vi "Read Method.vi"(11 "Filter in":refnum<class "Filter.lvclass">) -> (2 "Method":T1, 3 "Filter out":refnum<class "Filter.lvclass">)   [LabVIEW 2018, in "GLog.lvlib" / "Filter.lvclass"]
uses:
  Filter.lvclass
  Aggregation Method.ctl
  Filter.lvclass/Filter.ctl
  GLog.lvlib
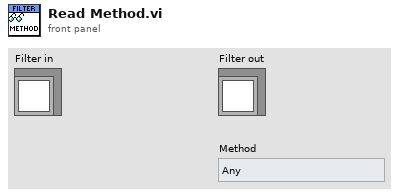
[diagram p1: front panel]
types:
  T1 = typedef "GLog.lvlib/Aggregation Method.ctl" = enum16{"Any", "Only", "All", "None"}
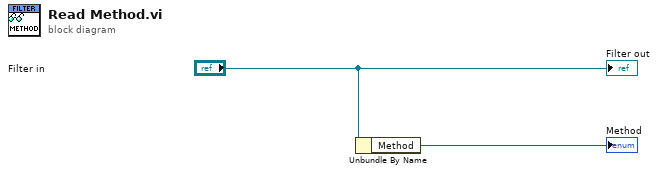
[diagram p0: block diagram]
diagram:
  n1 = Unbundle By Name("Filter in") -> ("Method"=→"Method":T1)
  "Filter out" <- "Filter in"
